vi "Test Parsing RE and DEC.vi"() -> ()   [LabVIEW 2021]
uses:
  typedefs/CC cluster RA and DEC.ctl
  Telescope/PRIME Telescope/PRIME Telescope.lvclass
panel:
  out "DEC String 3":string
  out "RA String 3":string
  out "RA and DEC 3":T1
  in  "DEC String 2":string
  in  "RA String 2":string
  out "RA and DEC 2":T1
  out "DEC String":string
  out "RA String":string
  in  "RA and DEC":T1
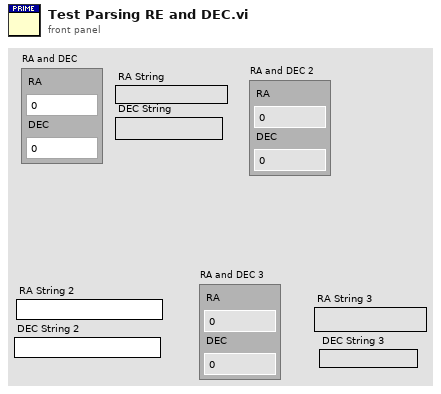
[diagram p1: front panel]
types:
  T1 = typedef "CC cluster RA and DEC.ctl" = cluster{"RA":dbl, "DEC":dbl}
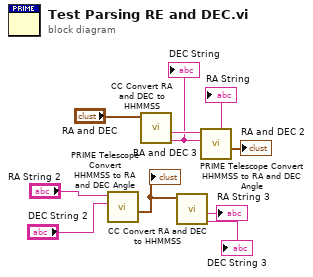
[diagram p0: block diagram]
diagram:
  n1 = call "PRIME Telescope Convert HHMMSS to RA and DEC Angle.vi"("Dec String"="DEC String 2", "RA String"="RA String 2") -> ("RA and DEC"=w3:T1)  [unwired: 7 in, 2 out]
  "RA and DEC 3" <- w3
  n2 = call "CC Convert RA and DEC to HHMMSS.vi"("RA and DEC"="RA and DEC") -> ("DEC String"=w7:string, "RA String"=w8:string)  [unwired: 7 in, 2 out]
  "RA String" <- w8
  "DEC String" <- w7
  n3 = call "CC Convert RA and DEC to HHMMSS.vi"("RA and DEC"=w3) -> ("DEC String"=→"DEC String 3":string, "RA String"=→"RA String 3":string)  [unwired: 7 in, 2 out]
  n4 = call "PRIME Telescope Convert HHMMSS to RA and DEC Angle.vi"("Dec String"=w7, "RA String"=w8) -> ("RA and DEC"=→"RA and DEC 2":T1)  [unwired: 7 in, 2 out]
